vi "FM Modulation Demo (Single tone) - Second(Phase-Locked Loop).vi"() -> ()   [LabVIEW 2013]
uses:
  <vilib>/addons/Modulation/Analog/MT Passband PLL.vi
  <vilib>/Waveform/WDTOps.llb/WDT Get Waveform Subset DBL.vi
  <vilib>/express/express analysis/Spectral/Block/exnSpectralBlock spectral measurements RMS poly.vi
  <vilib>/express/express analysis/Spectral/Block/exnSpectralBlock spectral measurements RMS DDT.vi
  <vilib>/express/express analysis/Spectral/XNode/ExpressSpectralMeasurementsBlockNode.xnode
  <vilib>/addons/Modulation/niAMT.lvlib
  <vilib>/Analysis/NI_AALPro.lvlib
panel:
  in  "WAV Sample Rate":dbl=44100.0 caption="dt"
  in  "Mod. Freq.":dbl=2000.0 caption="Frequency"
  in  "LPF Cut-Off":dbl=10000.0 caption="Lower Cut-Off"
  in  "AWGN (dB)":dbl(slide)=0.6 caption="Standard deviation" scale=-20.0..30.0
  out "Comparision":dynamicdata(graph)
  out "Baseband":dynamicdata(graph)
  out "FM FFT":dynamicdata(graph)
  out "FM Wave":dynamicdata(graph)
  out "Estimated freq":dbl=1.0
  in  "Carrier Amp.":dbl=1.0 caption="Amplitude"
  in  "stop":bool
  in  "Frequency Deviation":dbl(slide)=1.0 scale=0.0..5.0
  in  "Carrier Freq.":dbl=100000.0 caption="Frequency"
  out "After Rectifier":cluster{"f0":dbl, "df":dbl, "magnitude":dbl[]}(graph)
  # "FM Modulation"
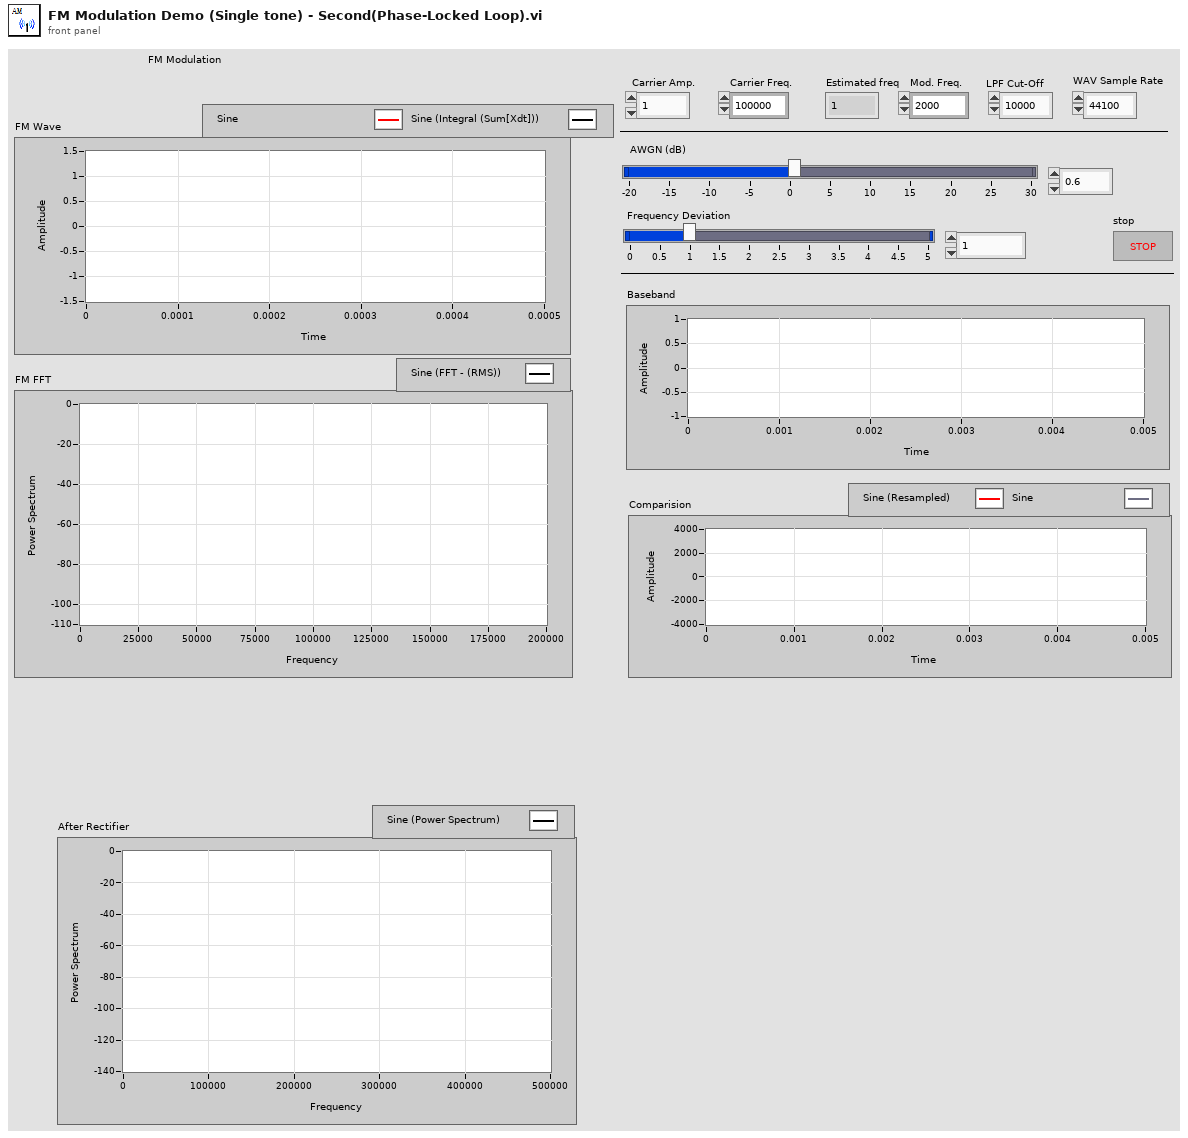
[diagram p1: front panel]
types:
  T1 = cluster{"averaging mode":u16, "weighting mode":u16, "number of averages":u32}
  T2 = cluster{"dB On (F)":bool, "unwrap phase (F)":bool, "convert to degree (F)":bool}
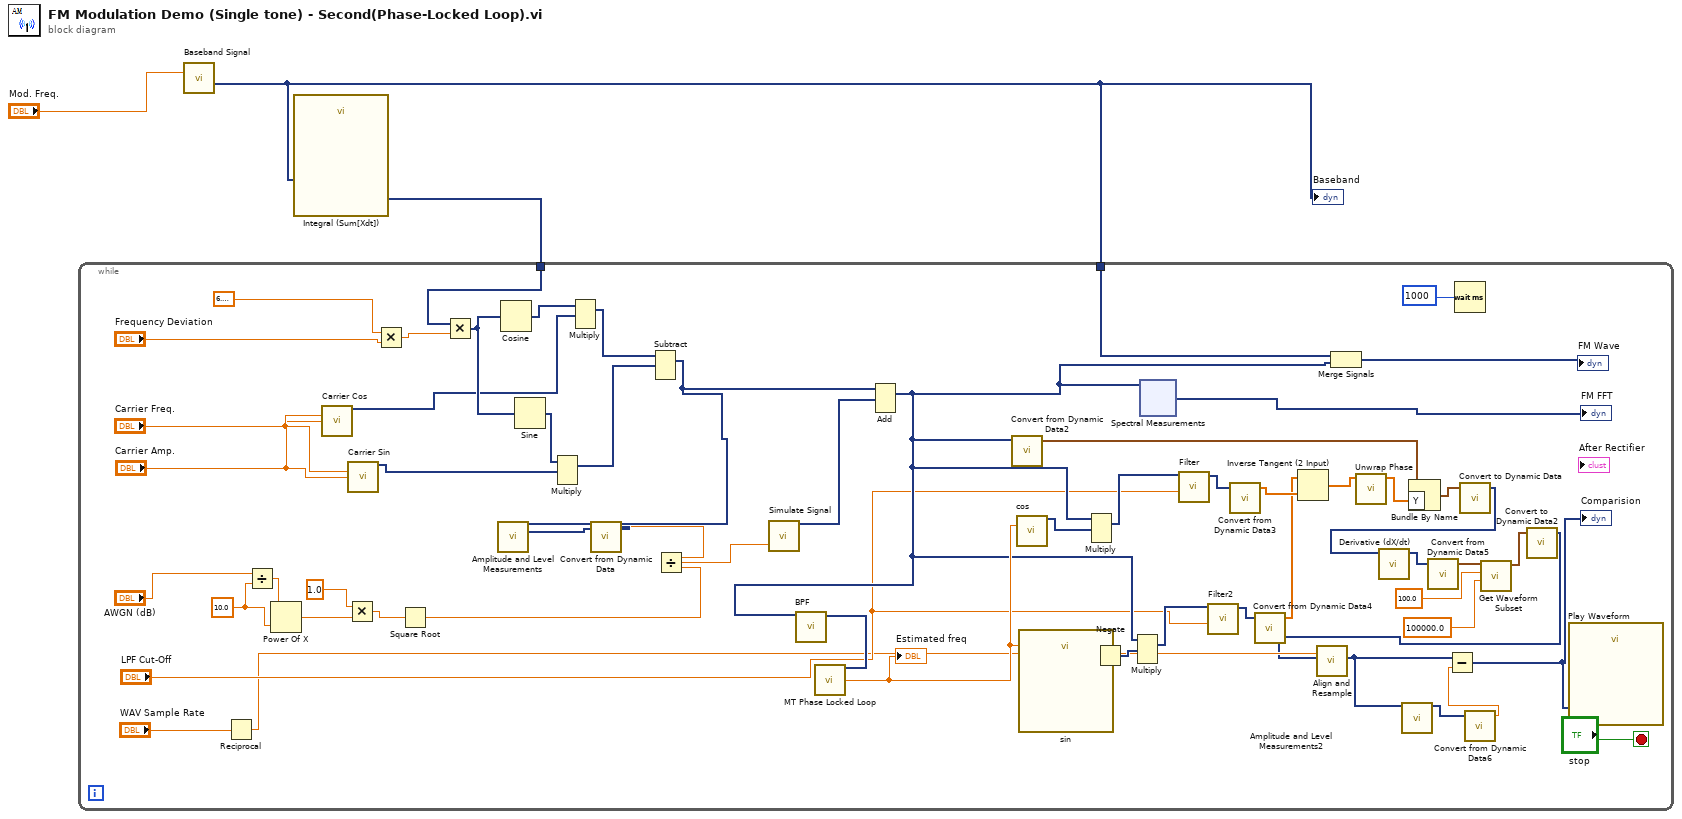
[diagram p0: block diagram]
diagram:
  n1 = call "Baseband Signal"("Frequency"="Mod. Freq.") -> ("Sine"=w2:dynamicdata)  [unwired: 13 in, 1 out]
  "Baseband" <- w2
  n2 = call "Integral (Sum[Xdt])"("Signals"=w2) -> ("Result"=w1:dynamicdata)  [unwired: 5 in, 1 out]
  n3 = while {
    tunnel: w2 -> [w41]
    tunnel: w1 -> [w45]
    stop <- "stop" stop-if-true
    w50 = 10.0
    n4 = Reciprocal(x="WAV Sample Rate") -> (1/x=w12:dbl)
    n5 = Divide(x="AWGN (dB)", y=w50) -> (x/y=w51:dbl)
    n6 = Power Of X(1:w50, 2:w51) -> (0:w49:dbl)
    n7 = call "Carrier Cos"("Frequency"="Carrier Freq.", "Amplitude"="Carrier Amp.") -> ("Sine"=w35:dynamicdata)  [unwired: 12 in, 1 out]
    n8 = Multiply(x=1.0, y=w49) -> (x*y=w57:dbl)
    n9 = call "Carrier Sin"("Frequency"="Carrier Freq.", "Amplitude"="Carrier Amp.") -> ("Sine"=w39:dynamicdata)  [unwired: 12 in, 1 out]
    n10 = Multiply(x=6.283185307179586, y="Frequency Deviation") -> (x*y=w46:dbl)
    n11 = Square Root(x=w57) -> (sqrt(x)=w55:dbl)
    n12 = Multiply(x=w45, y=w46) -> (x*y=w38:dynamicdata)
    n13 = Cosine(x=w38) -> (cos(x)=w36:dynamicdata)
    n14 = Sine(x=w38) -> (sin(x)=w37:dynamicdata)
    n15 = Multiply(1:w39, 2:w37) -> (0:w40:dynamicdata)  [unwired: 1 in, 1 out]
    n16 = Multiply(1:w35, 2:w36) -> (0:w34:dynamicdata)  [unwired: 1 in, 1 out]
    n17 = Subtract(1:w40, 2:w34) -> (0:w42:dynamicdata)  [unwired: 1 in, 1 out]
    n18 = call "Amplitude and Level Measurements"("Signals"=w42) -> ("RMS"=w60:dynamicdata)  [unwired: 13 in, 1 out]
    n19 = call "Convert from Dynamic Data"("Dynamic Data Type"=w60) -> ("Scalar"=w56:dbl)  [unwired: 3 in]
    n20 = Divide(x=w56, y=w55) -> (x/y=w48:dbl)
    n21 = call "Simulate Signal"("Standard deviation"=w48) -> ("DC with Gaussian Noise"=w54:dynamicdata)  [unwired: 13 in, 1 out]
    n22 = Add(1:w54, 2:w42) -> (0:w28:dynamicdata)  [unwired: 1 in, 1 out]
    n23 = call "BPF"("Signal"=w28) -> ("Filtered Signal"=w33:dynamicdata)  [unwired: 9 in, 1 out]
    n24 = call-poly <vilib>:"MT Phase Locked Loop.vi"("passband waveform"=w33) -> ("estimated carrier frequency (Hz)"=w31:dbl)  [unwired: 10 in, 4 out]
    "Estimated freq" <- w31
    n25 = call "Convert from Dynamic Data2"("Dynamic Data Type"=w28) -> ("Waveform"=w22:waveform(dbl))  [unwired: 3 in]
    n26 = call "cos"("Frequency"=w31) -> ("Sine"=w32:dynamicdata)  [unwired: 13 in, 1 out]
    n27 = call "sin"("Frequency"=w31) -> ("Sine"=w30:dynamicdata)  [unwired: 13 in, 1 out]
    n28 = Multiply(1:w32, 2:w28) -> (0:w27:dynamicdata)  [unwired: 1 in, 1 out]
    n29 = Negate(x=w30) -> (-x=w29:dynamicdata)
    n30 = Multiply(1:w29, 2:w28) -> (0:w26:dynamicdata)  [unwired: 1 in, 1 out]
    n31 = xnode "Spectral Measurements"("Signals"=w28) -> ("FFT - (RMS)"=→"FM FFT":dynamicdata)  [unwired: 1 in, 2 out]
    n32 = call "Filter"("Lower Cut-Off"="LPF Cut-Off", "Signal"=w27) -> ("Filtered Signal"=w24:dynamicdata)  [unwired: 8 in, 1 out]
    n33 = call "Filter2"("Lower Cut-Off"="LPF Cut-Off", "Signal"=w26) -> ("Filtered Signal"=w23:dynamicdata)  [unwired: 8 in, 1 out]
    n34 = call "Convert from Dynamic Data3"("Dynamic Data Type"=w24) -> ("Array"=w6:dbl[])  [unwired: 3 in]
    n35 = call "Convert from Dynamic Data4"("Dynamic Data Type"=w23) -> ("Array"=w5:dbl[])  [unwired: 3 in]
    n36 = Inverse Tangent (2 Input)(1:w6, 2:w5) -> (0:w4:dbl[])
    n37 = Merge Signals(w41, w28) -> (→"FM Wave":dynamicdata)
    n38 = call <vilib>:"Unwrap Phase.vi"("Phase"=w4) -> ("Unwrapped Phase"=w21:dbl[])  [unwired: 9 in, 1 out]
    n39 = Bundle By Name(cluster=w22, "Y"=w21) -> (w20:waveform(dbl))
    n40 = Wait (ms)(milliseconds to wait=1000) -> ()  [unwired: 1 out]
    n41 = call "Convert to Dynamic Data"("Waveform"=w20) -> ("Dynamic Data Type"=w19:dynamicdata)  [unwired: 3 in]
    n42 = call "Derivative (dX/dt)"("Signals"=w19) -> ("Result"=w18:dynamicdata)  [unwired: 5 in, 1 out]
    n43 = call "Convert from Dynamic Data5"("Dynamic Data Type"=w18) -> ("Waveform"=w17:waveform(dbl))  [unwired: 3 in]
    n44 = call-poly <vilib>:"Get Waveform Subset.vi"("duration"=100000.0, "start samples/time"=100.0, "waveform in"=w17) -> ("waveform out"=w14:waveform(dbl))  [unwired: 3 in, 3 out]
    n45 = call "Convert to Dynamic Data2"("Waveform"=w14) -> ("Dynamic Data Type"=w11:dynamicdata)  [unwired: 3 in]
    n46 = call "Align and Resample"("dt"=w12, "Signals"=w11) -> ("Resampled Signals"=w9:dynamicdata)  [unwired: 7 in, 2 out]
    n47 = call "Amplitude and Level Measurements2"("Signals"=w9) -> ("Mean (DC)"=w10:dynamicdata)  [unwired: 13 in, 1 out]
    n48 = call "Convert from Dynamic Data6"("Dynamic Data Type"=w10) -> ("Scalar"=w8:dbl)  [unwired: 3 in]
    n49 = Subtract(x=w9, y=w8) -> (x-y=w7:dynamicdata)
    "Comparision" <- w7
    n50 = call "Play Waveform"("Data"=w7) -> ()  [unwired: 18 in, 1 out]
  }
